vi "VerifPrevErrors.vi"(8 "error in (no error)":errorcluster, 11 "S4GUI in":refnum<class "S4GUI.lvclass">) -> (0 "error out":errorcluster, 3 "S4GUI out":refnum<class "S4GUI.lvclass">)   [LabVIEW 2018, in "S4GUI.lvclass"]
uses:
  S4GUI.lvclass
  S4GUI.lvclass/S4GUI.ctl
  Acquisition/Acquisition.lvclass
  Channel/Channel.lvclass
  StateMachine/State Machine.lvclass
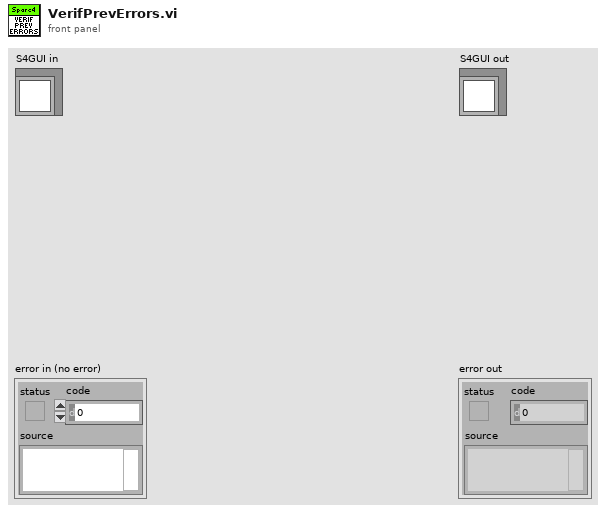
[diagram p1: front panel]
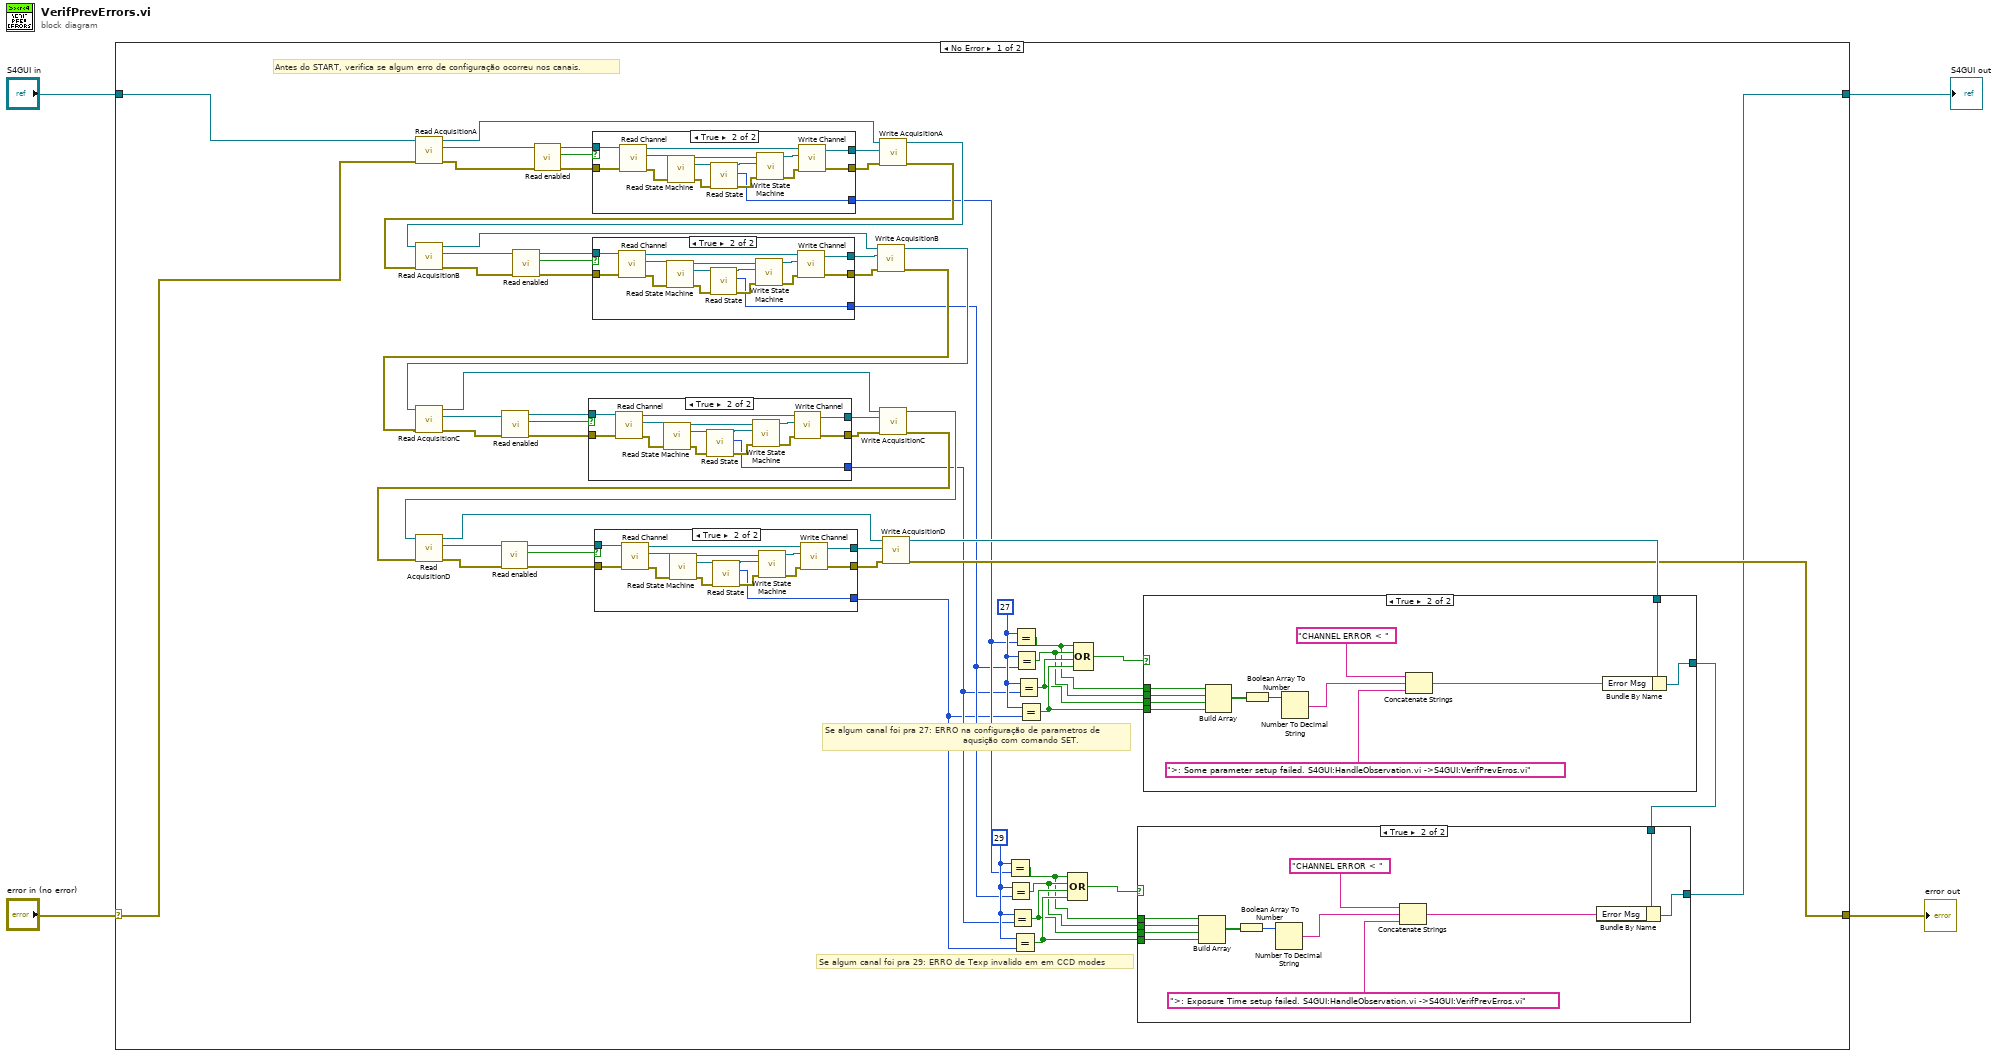
[diagram p0: block diagram]
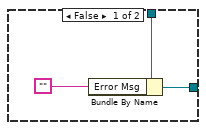
[diagram p3: hidden frame]
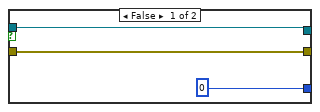
[diagram p4: hidden frame]
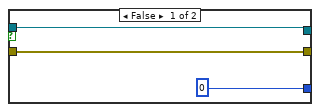
[diagram p5: hidden frame]
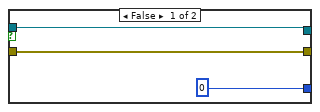
[diagram p6: hidden frame]
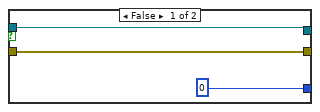
[diagram p7: hidden frame]
diagram:
  n1 = case shown="No Error" "error in (no error)" {
    selector: "error in (no error)" -> [w18 w166]
    tunnel: [w19 w166] -> w3
    tunnel: [w9 w165] -> w1
    tunnel: "S4GUI in" -> [w21 w165]
    frame No Error {
      w16 = 29 ("x")
      w26 = 27 ("x")
      # "Se algum canal foi pra 29: ERRO de Texp invalido em em CCD modes"
      # "Antes do START, verifica se algum erro de configuração ocorreu nos canais."
      # "Se algum canal foi pra 27: ERRO na configuração de parametros de\n                                              aqusição com comando SET."
      n2 = call-dynamic "Read AcquisitionA.vi"("error in (no error)"=w18, "S4ACS_GUI in"=w21) -> ("error out"=w52:errorcluster, "Acquisition.lvclass"=w53:refnum<class "Acquisition.lvclass">, "S4ACS_GUI out"=w63:refnum<class "S4GUI.lvclass">)  [unwired: 7 in]
      n3 = call-dynamic "Read enabled.vi"("error in (no error)"=w52, "Server in"=w53) -> ("error out"=w50:errorcluster, "enabled"=w49:bool, "Server out"=w51:refnum<class "Acquisition.lvclass">)  [unwired: 7 in]
      n4 = case shown="True" w49 {
        tunnel: w51 -> [w148 w164]
        tunnel: w50 -> [w147 w163]
        tunnel: [w148 w161] -> w64
        tunnel: [w147 w160] -> w62
        tunnel: [0 ("State") w150] -> w8
        frame False {
        }
        frame True {
          n5 = call-dynamic "Read Channel.vi"("error in (no error)"=w163, "Acquisition in"=w164) -> ("error out"=w159:errorcluster, "Channel.lvclass"=w158:refnum<class "Channel.lvclass">, "Acquisition out"=w162:refnum<class "Acquisition.lvclass">)  [unwired: 7 in]
          n6 = call-dynamic "Read State Machine.vi"("error in (no error)"=w159, "Device in"=w158) -> ("error out"=w152:errorcluster, "State Machine.lvclass"=w154:refnum<class "State Machine.lvclass">, "Device out"=w156:refnum<class "Channel.lvclass">)  [unwired: 7 in]
          n7 = call-dynamic "Read State.vi"("error in (no error)"=w152, "State Machine in"=w154) -> ("error out"=w151:errorcluster, "State"=w150:i32, "State Machine out"=w153:refnum<class "State Machine.lvclass">)  [unwired: 7 in]
          n8 = call-dynamic "Write State Machine.vi"("error in (no error)"=w151, "State Machine.lvclass"=w153, "Device in"=w156) -> ("error out"=w155:errorcluster, "Device out"=w157:refnum<class "Channel.lvclass">)  [unwired: 7 in]
          n9 = call-dynamic "Write Channel.vi"("error in (no error)"=w155, "Channel.lvclass"=w157, "Acquisition in"=w162) -> ("error out"=w160:errorcluster, "Acquisition out"=w161:refnum<class "Acquisition.lvclass">)  [unwired: 7 in]
        }
      }
      n10 = call-dynamic "Write AcquisitionA.vi"("error in (no error)"=w62, "Acquisition.lvclass"=w64, "S4ACS_GUI in"=w63) -> ("error out"=w59:errorcluster, "S4ACS_GUI out"=w58:refnum<class "S4GUI.lvclass">)  [unwired: 7 in]
      n11 = call "Read AcquisitionB.vi"("error in (no error)"=w59, "S4ACS_GUI in"=w58) -> ("error out"=w44:errorcluster, "Acquisition.lvclass"=w47:refnum<class "Acquisition.lvclass">, "S4ACS_GUI out"=w48:refnum<class "S4GUI.lvclass">)  [unwired: 7 in]
      n12 = call-dynamic "Read enabled.vi"("error in (no error)"=w44, "Server in"=w47) -> ("error out"=w43:errorcluster, "enabled"=w45:bool, "Server out"=w46:refnum<class "Acquisition.lvclass">)  [unwired: 7 in]
      n13 = case shown="True" w45 {
        tunnel: w46 -> [w130 w146]
        tunnel: w43 -> [w129 w145]
        tunnel: [w130 w143] -> w42
        tunnel: [w129 w142] -> w41
        tunnel: [0 ("State") w132] -> w7
        frame False {
        }
        frame True {
          n14 = call-dynamic "Read Channel.vi"("error in (no error)"=w145, "Acquisition in"=w146) -> ("error out"=w141:errorcluster, "Channel.lvclass"=w140:refnum<class "Channel.lvclass">, "Acquisition out"=w144:refnum<class "Acquisition.lvclass">)  [unwired: 7 in]
          n15 = call-dynamic "Read State Machine.vi"("error in (no error)"=w141, "Device in"=w140) -> ("error out"=w134:errorcluster, "State Machine.lvclass"=w136:refnum<class "State Machine.lvclass">, "Device out"=w138:refnum<class "Channel.lvclass">)  [unwired: 7 in]
          n16 = call-dynamic "Read State.vi"("error in (no error)"=w134, "State Machine in"=w136) -> ("error out"=w133:errorcluster, "State"=w132:i32, "State Machine out"=w135:refnum<class "State Machine.lvclass">)  [unwired: 7 in]
          n17 = call-dynamic "Write State Machine.vi"("error in (no error)"=w133, "State Machine.lvclass"=w135, "Device in"=w138) -> ("error out"=w137:errorcluster, "Device out"=w139:refnum<class "Channel.lvclass">)  [unwired: 7 in]
          n18 = call-dynamic "Write Channel.vi"("error in (no error)"=w137, "Channel.lvclass"=w139, "Acquisition in"=w144) -> ("error out"=w142:errorcluster, "Acquisition out"=w143:refnum<class "Acquisition.lvclass">)  [unwired: 7 in]
        }
      }
      n19 = call "Write AcquisitionB.vi"("error in (no error)"=w41, "Acquisition.lvclass"=w42, "S4ACS_GUI in"=w48) -> ("error out"=w57:errorcluster, "S4ACS_GUI out"=w56:refnum<class "S4GUI.lvclass">)  [unwired: 7 in]
      n20 = call-dynamic "Read AcquisitionC.vi"("error in (no error)"=w57, "S4ACS_GUI in"=w56) -> ("error out"=w39:errorcluster, "Acquisition.lvclass"=w40:refnum<class "Acquisition.lvclass">, "S4ACS_GUI out"=w61:refnum<class "S4GUI.lvclass">)  [unwired: 7 in]
      n21 = call-dynamic "Read enabled.vi"("error in (no error)"=w39, "Server in"=w40) -> ("error out"=w38:errorcluster, "enabled"=w36:bool, "Server out"=w37:refnum<class "Acquisition.lvclass">)  [unwired: 7 in]
      n22 = case shown="True" w36 {
        tunnel: w37 -> [w112 w128]
        tunnel: w38 -> [w111 w127]
        tunnel: [w112 w125] -> w35
        tunnel: [w111 w124] -> w34
        tunnel: [0 ("State") w114] -> w6
        frame False {
        }
        frame True {
          n23 = call-dynamic "Read Channel.vi"("error in (no error)"=w127, "Acquisition in"=w128) -> ("error out"=w123:errorcluster, "Channel.lvclass"=w122:refnum<class "Channel.lvclass">, "Acquisition out"=w126:refnum<class "Acquisition.lvclass">)  [unwired: 7 in]
          n24 = call-dynamic "Read State Machine.vi"("error in (no error)"=w123, "Device in"=w122) -> ("error out"=w116:errorcluster, "State Machine.lvclass"=w118:refnum<class "State Machine.lvclass">, "Device out"=w120:refnum<class "Channel.lvclass">)  [unwired: 7 in]
          n25 = call-dynamic "Read State.vi"("error in (no error)"=w116, "State Machine in"=w118) -> ("error out"=w115:errorcluster, "State"=w114:i32, "State Machine out"=w117:refnum<class "State Machine.lvclass">)  [unwired: 7 in]
          n26 = call-dynamic "Write State Machine.vi"("error in (no error)"=w115, "State Machine.lvclass"=w117, "Device in"=w120) -> ("error out"=w119:errorcluster, "Device out"=w121:refnum<class "Channel.lvclass">)  [unwired: 7 in]
          n27 = call-dynamic "Write Channel.vi"("error in (no error)"=w119, "Channel.lvclass"=w121, "Acquisition in"=w126) -> ("error out"=w124:errorcluster, "Acquisition out"=w125:refnum<class "Acquisition.lvclass">)  [unwired: 7 in]
        }
      }
      n28 = call-dynamic "Write AcquisitionC.vi"("error in (no error)"=w34, "Acquisition.lvclass"=w35, "S4ACS_GUI in"=w61) -> ("error out"=w55:errorcluster, "S4ACS_GUI out"=w54:refnum<class "S4GUI.lvclass">)  [unwired: 7 in]
      n29 = call-dynamic "Read AcquisitionD.vi"("error in (no error)"=w55, "S4ACS_GUI in"=w54) -> ("error out"=w31:errorcluster, "Acquisition.lvclass"=w33:refnum<class "Acquisition.lvclass">, "S4ACS_GUI out"=w60:refnum<class "S4GUI.lvclass">)  [unwired: 7 in]
      n30 = call-dynamic "Read enabled.vi"("error in (no error)"=w31, "Server in"=w33) -> ("error out"=w30:errorcluster, "enabled"=w29:bool, "Server out"=w32:refnum<class "Acquisition.lvclass">)  [unwired: 7 in]
      n31 = case shown="True" w29 {
        tunnel: w32 -> [w94 w110]
        tunnel: w30 -> [w93 w109]
        tunnel: [w94 w107] -> w28
        tunnel: [w93 w106] -> w27
        tunnel: [0 ("State") w96] -> w5
        frame False {
        }
        frame True {
          n32 = call-dynamic "Read Channel.vi"("error in (no error)"=w109, "Acquisition in"=w110) -> ("error out"=w105:errorcluster, "Channel.lvclass"=w104:refnum<class "Channel.lvclass">, "Acquisition out"=w108:refnum<class "Acquisition.lvclass">)  [unwired: 7 in]
          n33 = call-dynamic "Read State Machine.vi"("error in (no error)"=w105, "Device in"=w104) -> ("error out"=w98:errorcluster, "State Machine.lvclass"=w100:refnum<class "State Machine.lvclass">, "Device out"=w102:refnum<class "Channel.lvclass">)  [unwired: 7 in]
          n34 = call-dynamic "Read State.vi"("error in (no error)"=w98, "State Machine in"=w100) -> ("error out"=w97:errorcluster, "State"=w96:i32, "State Machine out"=w99:refnum<class "State Machine.lvclass">)  [unwired: 7 in]
          n35 = call-dynamic "Write State Machine.vi"("error in (no error)"=w97, "State Machine.lvclass"=w99, "Device in"=w102) -> ("error out"=w101:errorcluster, "Device out"=w103:refnum<class "Channel.lvclass">)  [unwired: 7 in]
          n36 = call-dynamic "Write Channel.vi"("error in (no error)"=w101, "Channel.lvclass"=w103, "Acquisition in"=w108) -> ("error out"=w106:errorcluster, "Acquisition out"=w107:refnum<class "Acquisition.lvclass">)  [unwired: 7 in]
        }
      }
      n37 = call-dynamic "Write AcquisitionD.vi"("error in (no error)"=w27, "Acquisition.lvclass"=w28, "S4ACS_GUI in"=w60) -> ("error out"=w19:errorcluster, "S4ACS_GUI out"=w20:refnum<class "S4GUI.lvclass">)  [unwired: 7 in]
      n38 = Equal?(x=w16, y=w8) -> (x = y?=w12:bool)
      n39 = Equal?(x=w16, y=w7) -> (x = y?=w13:bool)
      n40 = Equal?(x=w16, y=w6) -> (x = y?=w14:bool)
      n41 = Equal?(x=w16, y=w5) -> (x = y?=w15:bool)
      n42 = Equal?(x=w26, y=w8) -> (x = y?=w22:bool)
      n43 = Equal?(x=w26, y=w7) -> (x = y?=w23:bool)
      n44 = Equal?(x=w26, y=w6) -> (x = y?=w24:bool)
      n45 = Equal?(x=w26, y=w5) -> (x = y?=w25:bool)
      n46 = Compound Arithmetic op=OR(w12, w13, w14, w15) -> (w11:bool)
      n47 = Compound Arithmetic op=OR(w22, w23, w24, w25) -> (w17:bool)
      n48 = case shown="True" w17 {
        tunnel: w20 -> [w80 w92]
        tunnel: [w79 w91] -> w10
        tunnel: w25 -> [_ w85]
        tunnel: w24 -> [_ w86]
        tunnel: w23 -> [_ w87]
        tunnel: w22 -> [_ w88]
        frame False {
          n49 = Bundle By Name(cluster=w80, "Error Msg"="") -> (w79:refnum<class "S4GUI.lvclass">)
        }
        frame True {
          n50 = Build Array(w88, w87, w86, w85) -> (w90:bool[])
          n51 = Boolean Array To Number(Boolean array=w90) -> (number=w89:u32)
          n52 = Number To Decimal String(number=w89) -> (decimal integer string=w83:string)  [unwired: 1 in]
          n53 = Concatenate Strings("CHANNEL ERROR < " ("string"), w83, ">: Some parameter setup failed. S4GUI:HandleObservation.vi ->S4GUI:VerifPrevErros.vi" ("Error Msg")) -> (w82:string)
          n54 = Bundle By Name(cluster=w92, "Error Msg"=w82) -> (w91:refnum<class "S4GUI.lvclass">)
        }
      }
      n55 = case shown="True" w11 {
        tunnel: w10 -> [w65 w77]
        tunnel: [w65 w76] -> w9
        tunnel: w15 -> [_ w70]
        tunnel: w14 -> [_ w71]
        tunnel: w13 -> [_ w72]
        tunnel: w12 -> [_ w73]
        frame False {
        }
        frame True {
          n56 = Build Array(w73, w72, w71, w70) -> (w75:bool[])
          n57 = Boolean Array To Number(Boolean array=w75) -> (number=w74:u32)
          n58 = Number To Decimal String(number=w74) -> (decimal integer string=w68:string)  [unwired: 1 in]
          n59 = Concatenate Strings("CHANNEL ERROR < " ("string"), w68, ">: Exposure Time setup failed. S4GUI:HandleObservation.vi ->S4GUI:VerifPrevErros.vi" ("Error Msg")) -> (w67:string)
          n60 = Bundle By Name(cluster=w77, "Error Msg"=w67) -> (w76:refnum<class "S4GUI.lvclass">)
        }
      }
    }
    frame Error {
    }
  }
  "error out" <- w3
  "S4GUI out" <- w1
